vi "Initialize Default.vi"(8 "error in (no error)":errorcluster, 11 "Core Channels Configuration in":refnum<class "Channel Configuration.lvclass">) -> (0 "error out":errorcluster, 3 "Core Channels Configuration out":refnum<class "Channel Configuration.lvclass">)   [LabVIEW 2017, in "DSF Core.lvlib" / "Channel Configuration.lvclass"]
uses:
  Channel Configuration.lvclass
  Typedefs/Core Channel Configuration.ctl
  Typedefs/DSF Data Type.ctl
  Channel Configuration.lvclass/Channel Configuration.ctl
  DSF Core.lvlib
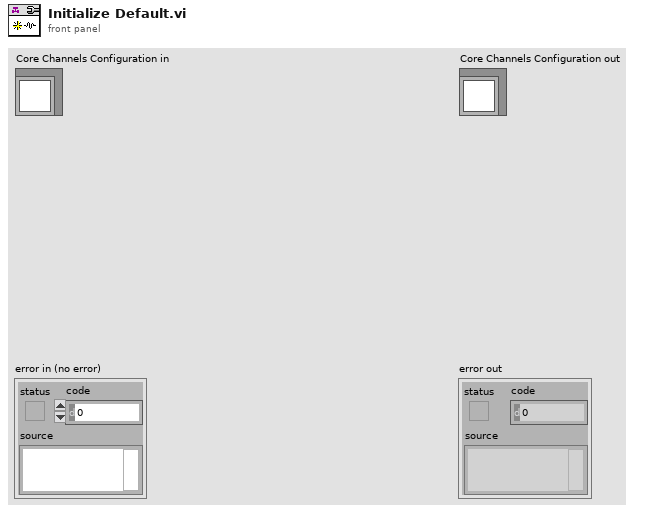
[diagram p1: front panel]
types:
  T1 = typedef "DSF Core.lvlib/Channel Configuration.lvclass/Core Channel Configuration.ctl" = cluster{"name":string, "units":string, "engine data type":T2, "string data type":T2, "string offset":u64}
  T2 = typedef "DSF Core.lvlib/DSF Data Type.ctl" = enum8{"Bool", "SGL", "DBL", "I8", "I16", "I32", "I64", "U8", "U16", "U32", "U64"}
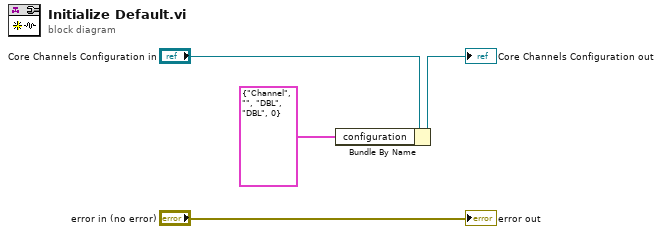
[diagram p0: block diagram]
diagram:
  n1 = Bundle By Name(cluster="Core Channels Configuration in", "configuration"=T1 {"name"="Channel", "units"="", "engine data type"=enum."DBL", "string data type"=enum."DBL", "string offset"=0}) -> (→"Core Channels Configuration out":refnum<class "Channel Configuration.lvclass">)
  "error out" <- "error in (no error)"
